vi "DUTtoNET.vi"(8 "error in (no error)":errorcluster, 11 "Engine Run-Time Data Cluster In":T1 {"Compiled Data"."Corruption Info DUT_Network"."Frame Infos Array"."CRC Index" min=-7 max=7; "Compiled Data"."Corruption Info DUT_Network"."Frame Infos Array"."DLC Length  Corruption Index" min=-8 max=8; "Compiled Data"."Corruption Info Network_DUT"."Frame Infos Array"."CRC Index" min=-7 max=7; "Compiled Data"."Corruption Info Network_DUT"."Frame Infos Array"."DLC Length  Corruption Index" min=-8 max=8; "Specified Channel Ref List Out" format="%.0x"; "Specified Channel Ref List In" format="%.0x"}) -> (0 "error out":errorcluster, 3 "Engine Run-Time Data Cluster Out":T1 {"Compiled Data"."Corruption Info DUT_Network"."Frame Infos Array"."CRC Index" min=-7 max=7; "Compiled Data"."Corruption Info DUT_Network"."Frame Infos Array"."DLC Length  Corruption Index" min=-8 max=8; "Compiled Data"."Corruption Info Network_DUT"."Frame Infos Array"."CRC Index" min=-7 max=7; "Compiled Data"."Corruption Info Network_DUT"."Frame Infos Array"."DLC Length  Corruption Index" min=-8 max=8; "Specified Channel Ref List Out" format="%.0x"; "Specified Channel Ref List In" format="%.0x"})   [LabVIEW 2018, in "CAN Gateway Engine.lvlib"]
uses:
  CAN Gateway Engine.lvlib
  Shared/CTLs/Runtime engine Data.ctl
  <vilib>/NI Veristand/Custom Device API/Custom Device Engine Event Ref.ctl
  <vilib>/NI Veristand/Custom Device API/Custom Device Item Ref.ctl
  Shared/CTLs/Compiled Data.ctl
  Shared/CTLs/Corruption Info.ctl
  Shared/CTLs/Frame.ctl
  Shared/CTLs/Signal_Data_Trigger.ctl
  <vilib>/xnet/xnet.llb/XNET Read (Frame CAN).vi
  <vilib>/xnet/xnet.llb/XNET Write (Frame CAN).vi
  <vilib>/NI Veristand/Custom Device API/Custom Device API.lvlib
  Shared/CAN Gateway Shared.lvlib
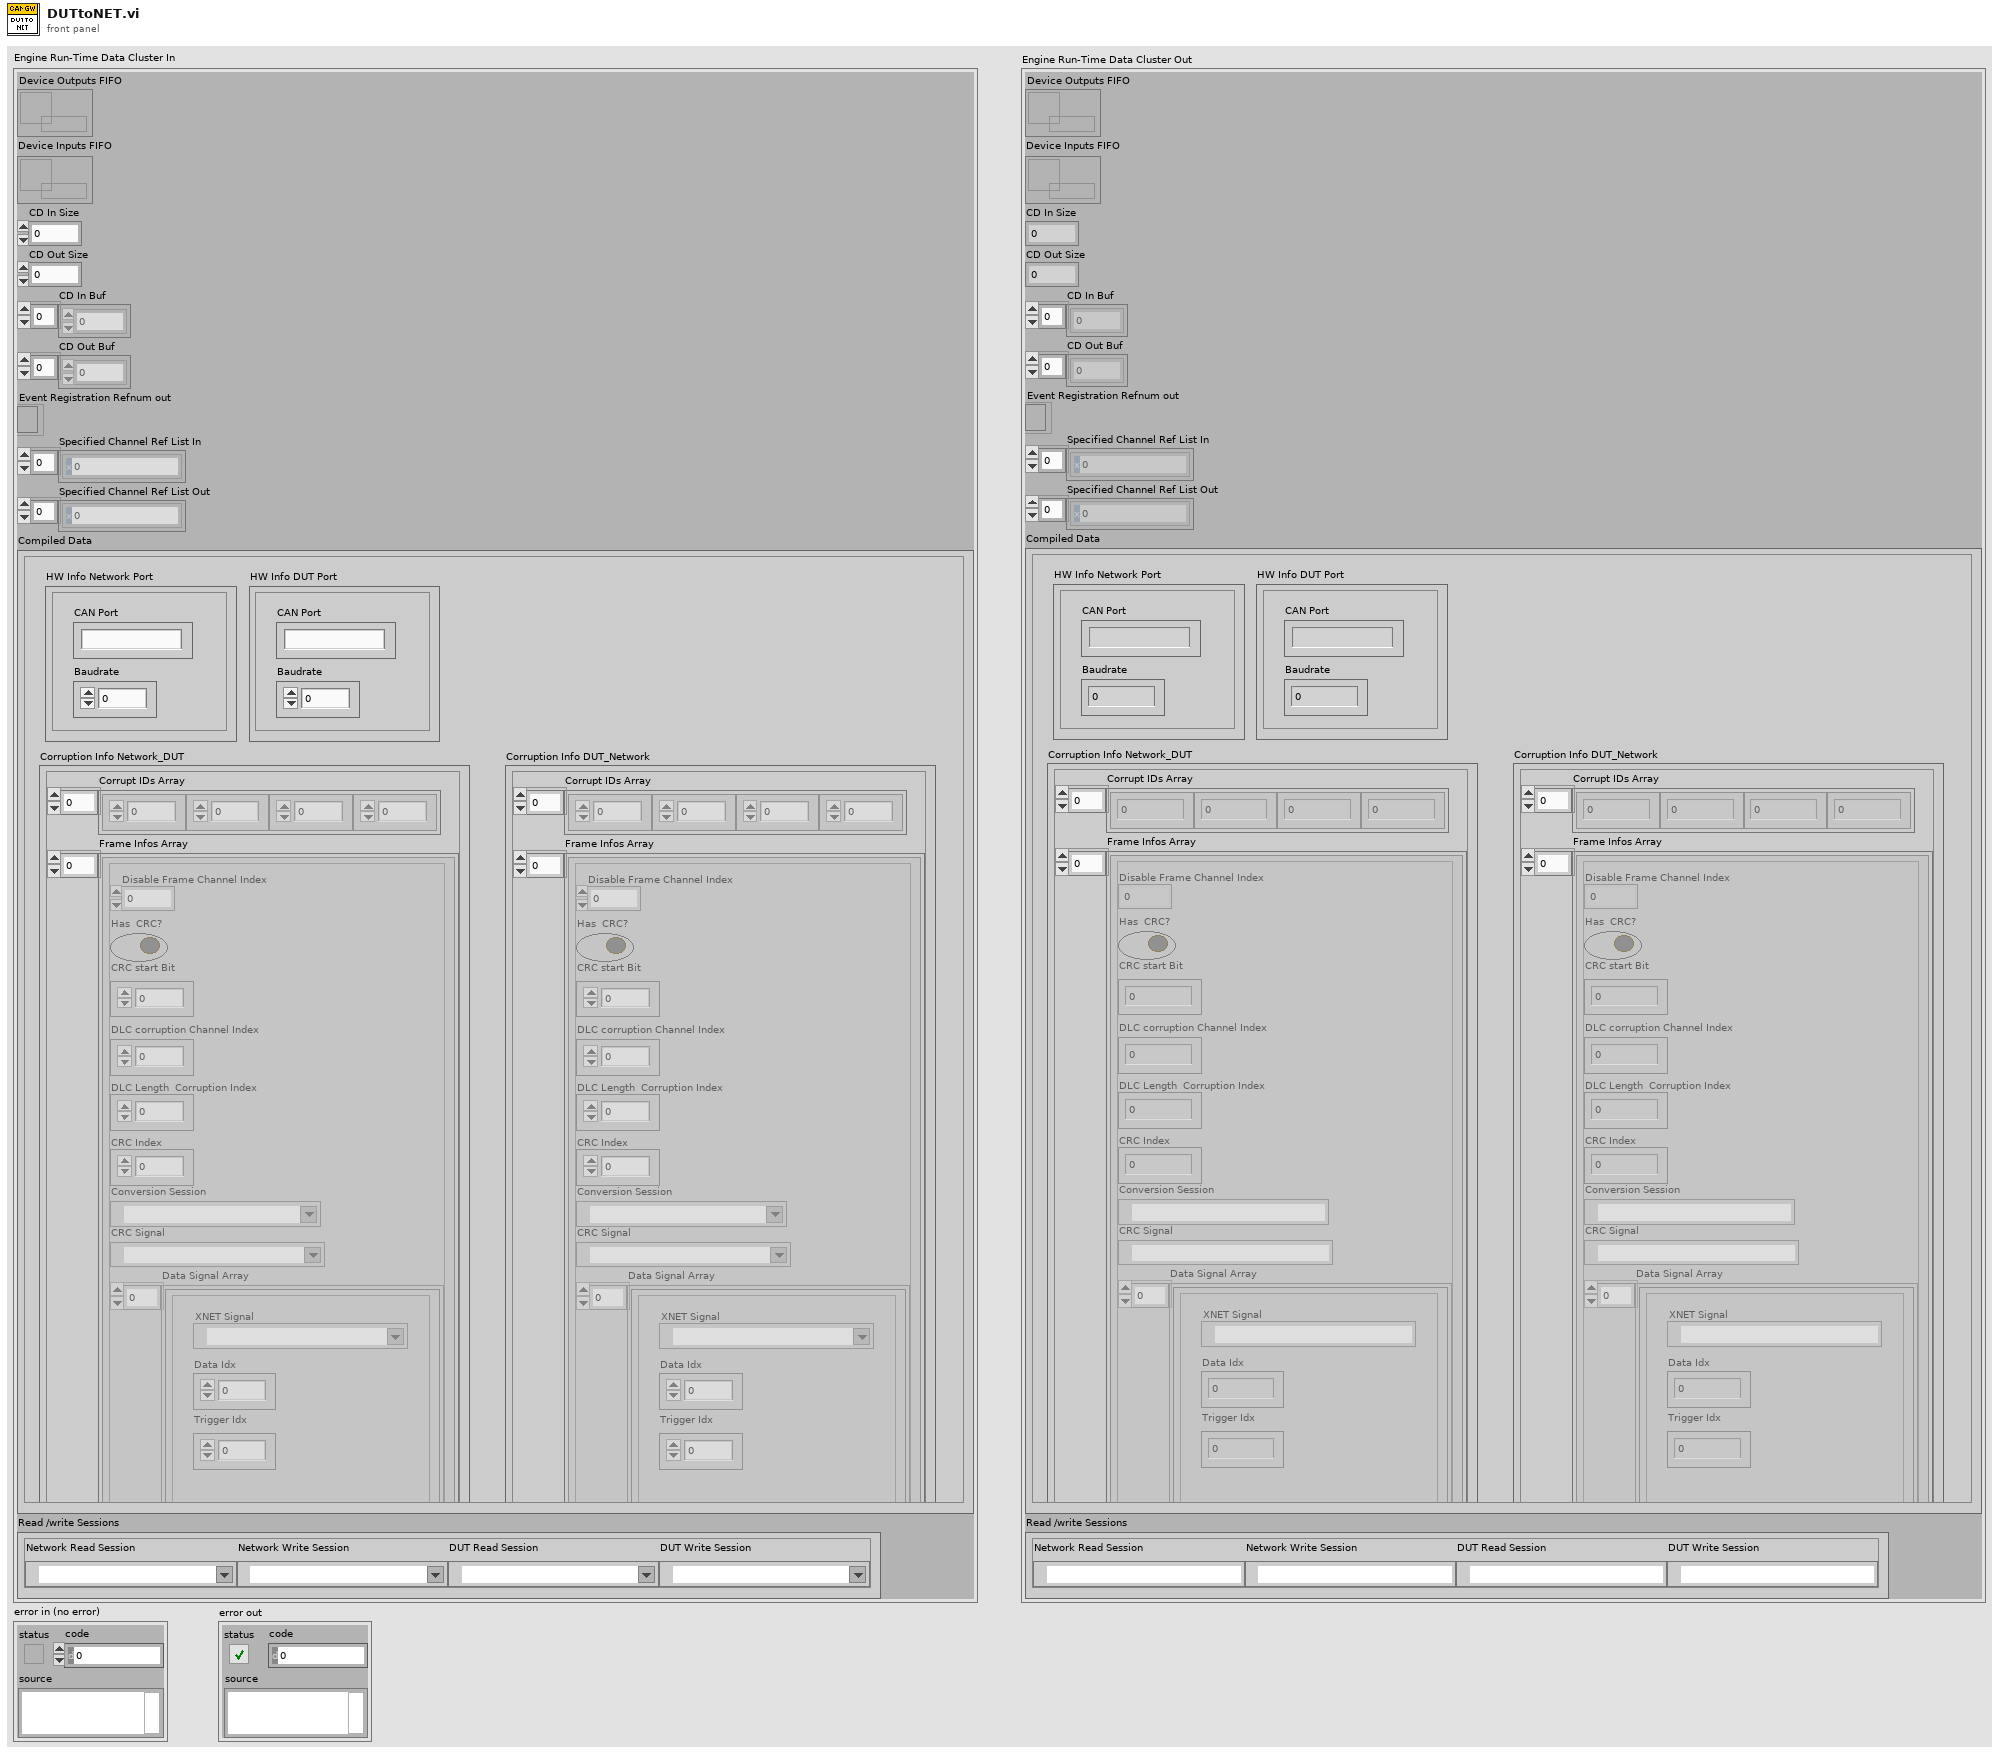
[diagram p1: front panel]
types:
  T1 = typedef "CAN Gateway Engine.lvlib/Runtime engine Data.ctl" = cluster{"Device Outputs FIFO":refnum<k33>, "Device Inputs FIFO":refnum<k33>, "CD In Size":i32, "CD Out Size":i32, "CD In Buf":dbl[], "CD Out Buf":dbl[], "Event Registration Refnum out":T2, "Specified Channel Ref List In":T3[], "Specified Channel Ref List Out":T3[], "Compiled Data":T4, "Read /write Sessions":cluster{"Network Read Session":refnum<k21>, "Network Write Session":refnum<k21>, "DUT Read Session":refnum<k21>, "DUT Write Session":refnum<k21>}}
  T2 = typedef "Custom Device API.lvlib/Custom Device Engine Event Ref.ctl" = refnum<event-registration>
  T3 = typedef "Custom Device API.lvlib/Custom Device Item Ref.ctl" = u64
  T4 = typedef "CAN Gateway Shared.lvlib/Compiled Data.ctl" = cluster{"HW Info Network Port":cluster{"CAN Port":string, "Baudrate":u64}, "HW Info DUT Port":cluster{"CAN Port":string, "Baudrate":u64}, "Corruption Info Network_DUT":T5, "Corruption Info DUT_Network":T5}
  T5 = typedef "CAN Gateway Shared.lvlib/Corruption Info.ctl" = cluster{"Corrupt IDs Array":u32[], "Frame Infos Array":T6[]}
  T6 = typedef "CAN Gateway Shared.lvlib/Frame.ctl" = cluster{"Disable Frame Channel Index":i32, "Has  CRC?":bool, "CRC start Bit":u32, "DLC corruption Channel Index":i32, "DLC Length  Corruption Index":i32, "CRC Index":i32, "Conversion Session":refnum<k21>, "CRC Signal":refnum<k21>, "Data Signal Array":T7[]}
  T7 = typedef "CAN Gateway Shared.lvlib/Signal_Data_Trigger.ctl" = cluster{"XNET Signal":refnum<k21>, "Data Idx":u32, "Trigger Idx":u32}
  T8 = typedef "XNET Frame CAN.ctl" = cluster{"timestamp":timestamp, "payload":u8[], "identifier":u32, "type":T9, "extended?":bool, "echo?":bool}
  T9 = typedef "XNET Frame Type CAN.ctl" = u8
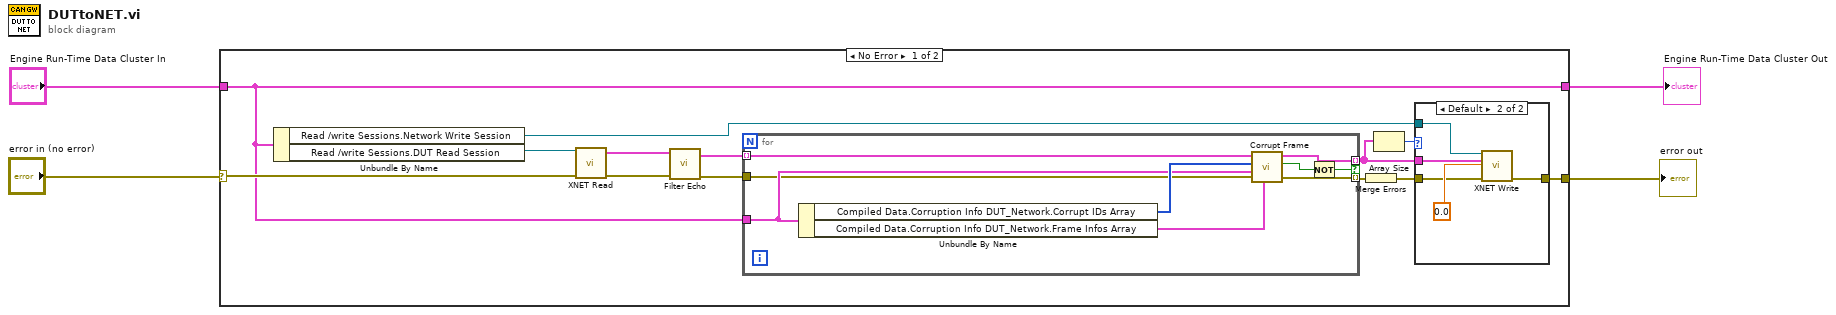
[diagram p0: block diagram]
diagram:
  n1 = case shown="No Error" "error in (no error)" {
    selector: "error in (no error)" -> [w16 w34]
    tunnel: [w11 w34] -> w3
    tunnel: "Engine Run-Time Data Cluster In" -> [w15 w33]
    tunnel: [w15 w33] -> w1
    frame No Error {
      n2 = Unbundle By Name(w15) -> ("Read /write Sessions.Network Write Session"=w14:refnum<k21>, "Read /write Sessions.DUT Read Session"=w17:refnum<k21>)
      n3 = call-poly <vilib>:"XNET Read.vi"("session in"=w17, "error in (no error)"=w16) -> ("data"=w10:T8[], "error out"=w7:errorcluster)  [unwired: 10 in, 2 out]
      n4 = call "Filter Echo.vi"("error in (no error)"=w7, "data in"=w10) -> ("error out"=w9:errorcluster, "data out"=w8:T8[])  [unwired: 8 in]
      n5 = for {
        tunnel: w8 -> [w30] mode=indexing
        tunnel: w15 -> [w31]
        tunnel: w9 -> [w29]
        tunnel: [w27] -> w13 mode=indexing
        tunnel: [w26] -> w5 mode=indexing if=w25
        n6 = Unbundle By Name(w31) -> ("Compiled Data.Corruption Info DUT_Network.Corrupt IDs Array"=w32:u32[], "Compiled Data.Corruption Info DUT_Network.Frame Infos Array"=w28:T6[])
        n7 = call "Corrupt Frame.vi"("Frame Infos Array"=w28, "error in (no error)"=w29, "Engine Run-Time Data Cluster In"=w31, "Corrupt IDs Array"=w32, "CAN frame"=w30) -> ("error out"=w27:errorcluster, "Disable Frame"=w24:bool, "Frame Data"=w26:T8)  [unwired: 4 in]
        n8 = Not(x=w24) -> (.not. x?=w25:bool)
      }
      n9 = Merge Errors(w13) -> (w12:errorcluster)
      n10 = Array Size(array=w5) -> (size(s)=w6:i32)
      n11 = case shown="Default" w6 {
        tunnel: w14 -> [_ w23]
        tunnel: w5 -> [_ w22]
        tunnel: w12 -> [w18 w20]
        tunnel: [w18 w19] -> w11
        frame 0 {
        }
        frame Default {
          n12 = call-poly <vilib>:"XNET Write.vi"("session in"=w23, "data"=w22, "timeout (10)"=0.0, "error in (no error)"=w20) -> ("error out"=w19:errorcluster)  [unwired: 10 in, 1 out]
        }
      }
    }
    frame Error {
    }
  }
  "error out" <- w3
  "Engine Run-Time Data Cluster Out" <- w1
